vi "FlatToRichnidaqmx_grpc_WriteDigitalLinesRequest.vi"(5 "OutputClusterType":T1, 11 "InputCluster":T3) -> (3 "OutputCluster":T1)   [LabVIEW 2021, in "NI DAQmx_server.lvlib"]
uses:
  NI DAQmx_server.lvlib
  nidaqmx_grpc_WriteDigitalLinesRequest_Flat.ctl
  nidevice_grpc_Session_Flat.ctl
  nidaqmx_grpc_GroupBy.ctl
  nidaqmx_grpc_WriteDigitalLinesRequest.ctl
  nidevice_grpc_Session_session/nidevice_grpc_Session_session.lvclass
  nidaqmx_grpc_WriteDigitalLinesRequest_data_layout_enum/nidaqmx_grpc_WriteDigitalLinesRequest_data_layout_enum.lvclass
  nidevice_grpc_Session.ctl
  nidevice_grpc_Session_session/nidevice_grpc_Session_session.lvclass/nidevice_grpc_Session_session.ctl
  nidaqmx_grpc_WriteDigitalLinesRequest_data_layout_enum/nidaqmx_grpc_WriteDigitalLinesRequest_data_layout_enum.lvclass/nidaqmx_grpc_WriteDigitalLinesRequest_data_layout_enum.ctl
  nidevice_grpc_Session_session/Setname.vi
  nidevice_grpc_Session_session/Setid.vi
  nidevice_grpc_Session_session/GetFieldFromProtobufIndexnidevice_grpc_Session_session.vi
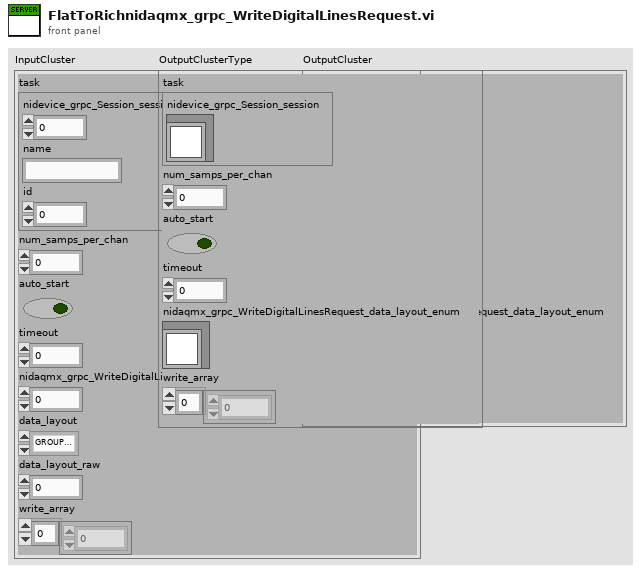
[diagram p1: front panel]
types:
  T1 = typedef "NI DAQmx_server.lvlib/nidaqmx_grpc_WriteDigitalLinesRequest.ctl" = cluster{"task":T2, "num_samps_per_chan":i32, "auto_start":bool, "timeout":dbl, "nidaqmx_grpc_WriteDigitalLinesRequest_data_layout_enum":refnum<class "nidaqmx_grpc_WriteDigitalLinesRequest_data_layout_enum.lvclass">, "write_array":u8[]}
  T2 = typedef "NI DAQmx_server.lvlib/nidevice_grpc_Session.ctl" = cluster{"nidevice_grpc_Session_session":refnum<class "nidevice_grpc_Session_session.lvclass">}
  T3 = typedef "NI DAQmx_server.lvlib/nidaqmx_grpc_WriteDigitalLinesRequest_Flat.ctl" = cluster{"task":T4, "num_samps_per_chan":i32, "auto_start":bool, "timeout":dbl, "nidaqmx_grpc_WriteDigitalLinesRequest_data_layout_enum_selected_index":i32, "data_layout":T5, "data_layout_raw":i32, "write_array":u8[]}
  T4 = typedef "NI DAQmx_server.lvlib/nidevice_grpc_Session_Flat.ctl" = cluster{"nidevice_grpc_Session_session_selected_index":i32, "name":string, "id":u32}
  T5 = typedef "NI DAQmx_server.lvlib/nidaqmx_grpc_GroupBy.ctl" = enum32{"GROUP_BY_GROUP_BY_CHANNEL", "GROUP_BY_GROUP_BY_SCAN_NUMBER"}
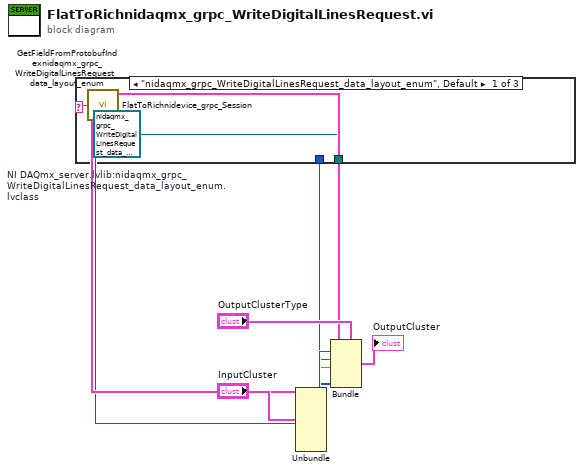
[diagram p0: block diagram]
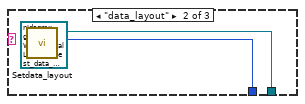
[diagram p2: hidden frame]
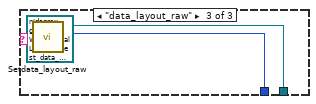
[diagram p3: hidden frame]
diagram:
  n1 = Unbundle "Unbundle"("InputCluster") -> ("task"=w11:T4, "num_samps_per_chan"=w9:i32, "auto_start"=w8:bool, "timeout"=w7:dbl, "nidaqmx_grpc_WriteDigitalLinesRequest_data_layout_enum_selected_index"=w6:i32, "data_layout"=w3:T5, "data_layout_raw"=w2:i32, "write_array"=w1:u8[])
  n2 = call "GetFieldFromProtobufIndexnidaqmx_grpc_WriteDigitalLinesRequest_data_layout_enum.vi"("protobuf index"=w6) -> ("oneof field name"=w5:string)
  n3 = case "nidaqmx_grpc_WriteDigitalLinesRequest_data_layout_enum" shown="\"nidaqmx_grpc_WriteDigitalLinesRequest_data_layout_enum\", Default" w5 {
    tunnel: [w15 w17 w20] -> w4
    tunnel: w3 -> [_ w18 _]
    tunnel: w2 -> [_ _ w21]
    frame "nidaqmx_grpc_WriteDigitalLinesRequest_data_layout_enum", Default {
      w15 = refnum<class "nidaqmx_grpc_WriteDigitalLinesRequest_data_layout_enum.lvclass"> refnum  # NI DAQmx_server.lvlib:nidaqmx_grpc_WriteDigitalLinesRequest_data_layout_enum.lvclass
    }
    frame "data_layout" {
      n4 = call "Setdata_layout.vi"("Set_Val"=w18, "OneOfTemplate in"=refnum<class "nidaqmx_grpc_WriteDigitalLinesRequest_data_layout_enum.lvclass"> refnum) -> ("OneOfTemplate out"=w17:refnum<class "nidaqmx_grpc_WriteDigitalLinesRequest_data_layout_enum.lvclass">)  [unwired: 8 in, 1 out]
    }
    frame "data_layout_raw" {
      n5 = call "Setdata_layout_raw.vi"("Set_Val"=w21, "OneOfTemplate in"=refnum<class "nidaqmx_grpc_WriteDigitalLinesRequest_data_layout_enum.lvclass"> refnum) -> ("OneOfTemplate out"=w20:refnum<class "nidaqmx_grpc_WriteDigitalLinesRequest_data_layout_enum.lvclass">)  [unwired: 8 in, 1 out]
    }
  }
  n6 = call "FlatToRichnidevice_grpc_Session.vi"("InputCluster"=w11) -> ("OutputCluster"=w10:T2)  [unwired: 10 in]
  n7 = Bundle "Bundle"(cluster="OutputClusterType", "task"=w10, "num_samps_per_chan"=w9, "auto_start"=w8, "timeout"=w7, "nidaqmx_grpc_WriteDigitalLinesRequest_data_layout_enum"=w4, "write_array"=w1) -> (→"OutputCluster":T1)
